vi "Boxcar filter.vi"(1 "Initialize":bool, 2 "Filter Size":i32, 3 "Filter Input":dbl format="%.2f") -> (0 "Filter Output":dbl format="%.2f")   [LabVIEW 2016]
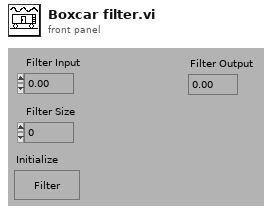
[diagram p1: front panel]
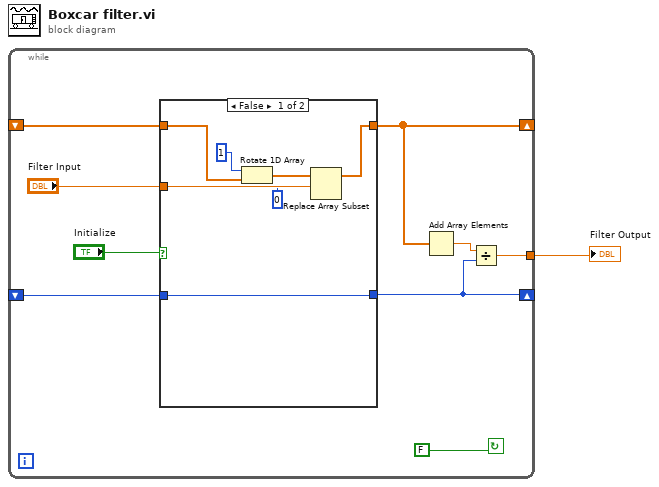
[diagram p0: block diagram]
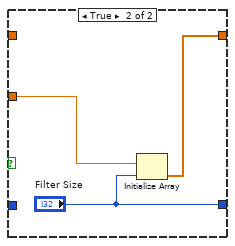
[diagram p2: hidden frame]
diagram:
  n1 = while {
    tunnel: [w4] -> w1
    shift-left: _ -> [w3]
    shift-right: [w5] -> _
    shift-left: _ -> [w2]
    shift-right: [w7] -> _
    stop <- FALSE continue-if-true
    n2 = case shown="False" "Initialize" {
      tunnel: "Filter Input" -> [w12 w20]
      tunnel: [w14 w19] -> w7
      tunnel: [w17 "Filter Size"] -> w5
      tunnel: w3 -> [w17 _]
      tunnel: w2 -> [w16 _]
      frame False {
        n3 = Rotate 1D Array(1:w16, 2:1) -> (0:w13:dbl[])
        n4 = Replace Array Subset(array=w13, new element=w12, index=0) -> (w14:dbl[])
      }
      frame True {
        n5 = Initialize Array(w20, "Filter Size") -> (w19:dbl[])
      }
    }
    n6 = Add Array Elements(numeric array=w7) -> (sum=w6:dbl)
    n7 = Divide(x=w6, y=w5) -> (x/y=w4:dbl)
  }
  "Filter Output" <- w1
